vi "Handle Camera Configuration.vi"(9 "CameraNameRef":refnum<vi>, 10 "Camera File Name":string="Camera", 11 "ClusterRef":refnum<vi>) -> ()   [LabVIEW 2016]
uses:
  <vilib>/Utility/config.llb/NI_LVConfig.lvlib
  <vilib>/Rock Robotics/Network Tables/Make Table Operation.ctl
  <vilib>/Utility/config.llb/Read Key (I32).vi
  <vilib>/Utility/config.llb/Read Key (String).vi
  <vilib>/Utility/config.llb/Write Key (I32).vi
  <vilib>/Utility/config.llb/Write Key (String).vi
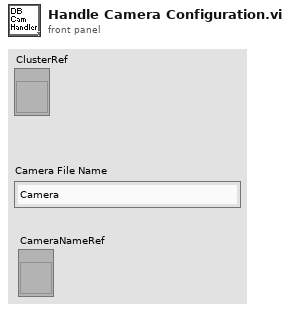
[diagram p1: front panel]
types:
  T1 = typedef "WPI_CameraDevRef.ctl" = cluster{"Camera Address":string, "CameraStatus":errorcluster}
  T2 = typedef "NI_LVConfig.lvlib/Config Data RefNum.ctl" = refnum<k1>
  T3 = cluster{"value":i32, "value":i32, "index":i32, bool}
  T4 = typedef "Make Table Operation.ctl" = enum16{"Get or Add Field", "Get Field or Add Temp", "Replace Temp ID", "Get Field ID - No Add", "Get Table Field IDs", "Get Field ID Info", "Move Field to Temp", "Validate", "Remove Field", "Remove All"}
  T5 = cluster{"Frame Rate":i32, "Compression":i32, "Size":u16, "DB Camera Config":bool}
  T6 = typedef "Field ID.ctl" = i32
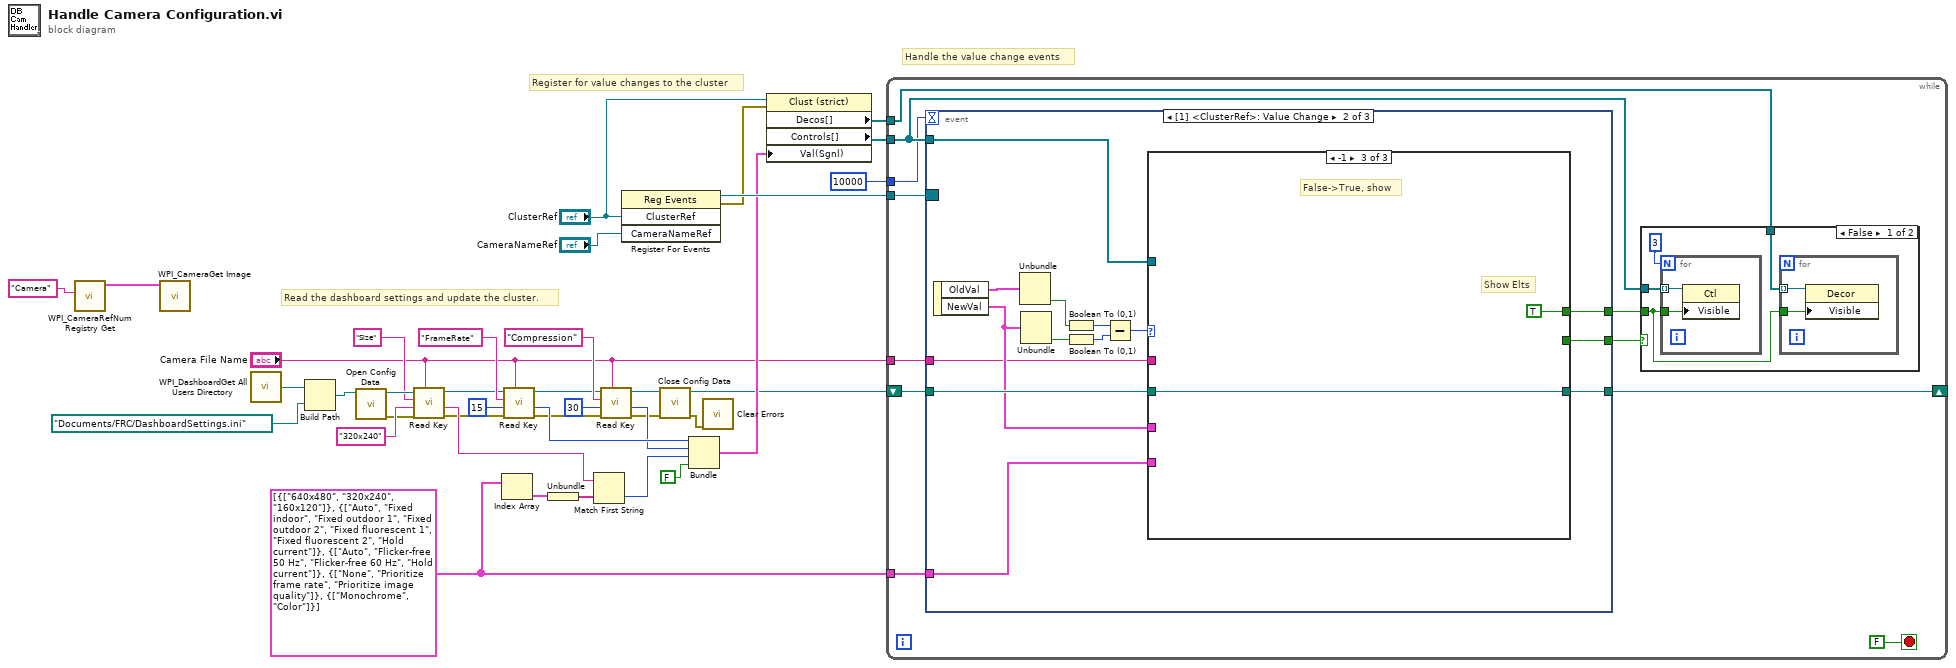
[diagram p0: block diagram]
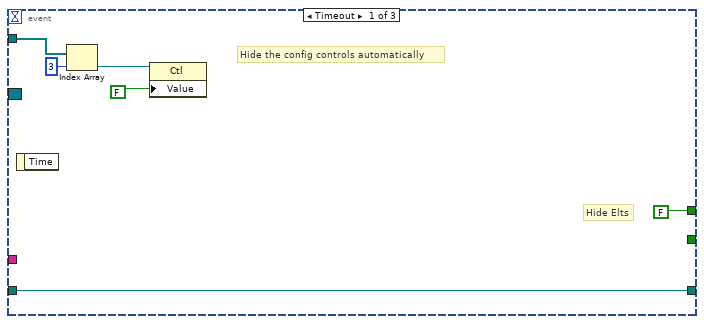
[diagram p3: hidden frame]
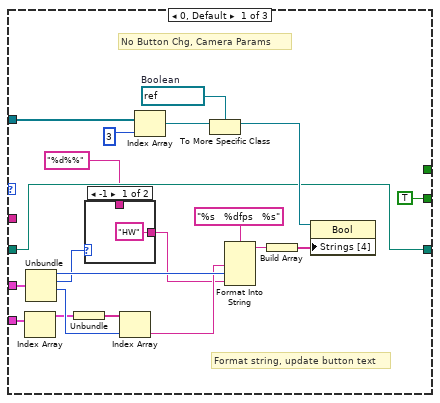
[diagram p4: hidden frame]
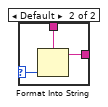
[diagram p5: hidden frame]
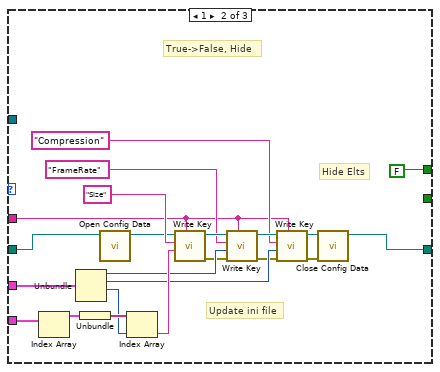
[diagram p6: hidden frame]
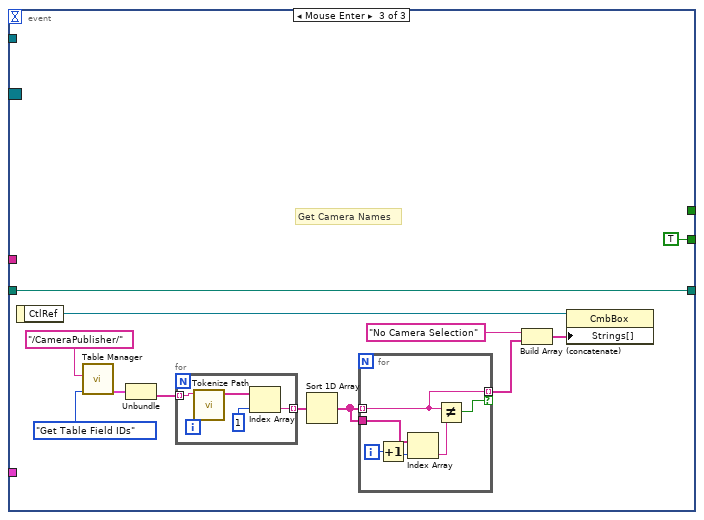
[diagram p7: hidden frame]
diagram:
  w17 = cluster{string[]}[] [{["640x480", "320x240", "160x120"]}, {["Auto", "Fixed indoor", "Fixed outdoor 1", "Fixed outdoor 2", "Fixed fluorescent 1", "Fixed fluorescent 2", "Hold current"]}, {["Auto", "Flicker-free 50 Hz", "Flicker-free 60 Hz", "Hold current"]}, {["None", "Prioritize frame rate", "Prioritize image quality"]}, {["Monochrome", "Color"]}]
  # "Handle the value change events"
  # "Register for value changes to the cluster"
  # "Read the dashboard settings and update the cluster."
  n1 = call <vilib>:"WPI_CameraRefNum Registry Get.vi"("refnum name"="Camera") -> ("CameraDevRef"=w1:T1)  [unwired: 9 in, 1 out]
  n2 = call <vilib>:"WPI_CameraGet Image.vi"("CameraDevRef"=w1) -> ()  [unwired: 8 in, 3 out]
  n3 = call <vilib>:"WPI_DashboardGet All Users Directory.vi"() -> ("All User Path"=w35:path)
  n4 = Build Path(base path=w35, name or relative path=path "Documents/FRC/DashboardSettings.ini") -> (appended path=w34:path)
  n5 = call <vilib>:"Open Config Data.vi"("configuration file path"=w34) -> ("error out"=w10:errorcluster, "refnum"=w33:T2)  [unwired: 8 in, 1 out]
  n6 = call-poly <vilib>:"Read Key.vi"("section"="Camera File Name", "error in (no error)"=w10, "default value"="320x240", "key"="Size", "refnum"=w33) -> ("error out"=w9:errorcluster, "value"=w21:string, "refnum out"=w25:T2)  [unwired: 1 in, 3 out]
  n7 = Index Array(array=w17) -> (element=w23:cluster{string[]})  [unwired: 1 in]
  n8 = call-poly <vilib>:"Read Key.vi"("section"="Camera File Name", "error in (no error)"=w9, "default value"=15, "key"="FrameRate", "refnum"=w25) -> ("error out"=w8:errorcluster, "value"=w19:i32, "refnum out"=w24:T2)  [unwired: 4 out]
  n9 = Unbundle(w23) -> (w22:string[])
  n10 = Match First String(2:w22, 3:w21) -> (0:w20:i32)  [unwired: 1 out]
  n11 = call-poly <vilib>:"Read Key.vi"("section"="Camera File Name", "error in (no error)"=w8, "default value"=30, "key"="Compression", "refnum"=w24) -> ("error out"=w5:errorcluster, "value"=w18:i32, "refnum out"=w7:T2)  [unwired: 4 out]
  n12 = register-events("ClusterRef", "CameraNameRef") -> (reference out=w38:refnum<event-registration>, error out=w15:errorcluster)  [unwired: 2 in]
  n13 = call <vilib>:"Close Config Data.vi"("error in (no error)"=w5, "refnum"=w7) -> ("error out"=w4:errorcluster, "file path"=w6:path)  [unwired: 1 in, 7 out]
  n14 = Bundle("value"=w19, "value"=w18, "index"=w20, FALSE) -> (w14:T3)  [unwired: 1 out]
  n15 = call <vilib>:"Clear Errors.vi"("error in (no error)"=w4) -> ()  [unwired: 5 in, 2 out]
  n16 = property class="Clust (strict)"(reference="ClusterRef", error in=w15, "Val(Sgnl)"=w14) -> ("Decos[]"=w12:refnum<vi>[], "Controls[]"=w36:refnum<vi>[])  [unwired: 2 out]
  n17 = while {
    tunnel: w38 -> [w49]
    tunnel: w36 -> [w41]
    shift-right: [w47] -> _
    shift-left: w6 -> [w48]
    tunnel: w17 -> [w46]
    tunnel: "Camera File Name" -> [w44]
    tunnel: w12 -> [w40]
    tunnel: 10000 -> [w39]
    stop <- FALSE stop-if-true
    n18 = event shown="[1] <ClusterRef>: Value Change" {
      selector: w49 -> [_ _ _]
      dyn-events: _ -> [_ _ _]
      timeout: w39 -> [_ _ _]
      tunnel: w48 -> [w62 w71 w135]
      tunnel: [w62 w67 w135] -> w47
      tunnel: w46 -> [_ w69 _]
      tunnel: w41 -> [w61 w68 _]
      tunnel: w44 -> [_ w66 _]
      tunnel: [FALSE w65 _] -> w42
      tunnel: [_ w64 TRUE] -> w43
      event Timeout {
        # "Hide Elts"
        # "Hide the config controls automatically"
        n19 = event-data() -> ()  [unwired: 1 in, 1 out]
        n20 = Index Array(array=w61, index=3) -> (element=w59:refnum<vi>)
        n21 = property class="Ctl"(reference=w59, "Value"=FALSE) -> ()  [unwired: 1 in, 2 out]
      }
      event Value Change {
        n22 = event-data() -> ("OldVal"=w73:T5, "NewVal"=w70:T5)  [unwired: 1 in]
        n23 = Unbundle(w73) -> ("DB Camera Config"=w77:bool)  [unwired: 3 out]
        n24 = Unbundle(w70) -> ("DB Camera Config"=w76:bool)  [unwired: 3 out]
        n25 = Boolean To (0,1)(Boolean=w77) -> (0, 1=w74:i16)
        n26 = Boolean To (0,1)(Boolean=w76) -> (0, 1=w75:i16)
        n27 = Subtract(x=w74, y=w75) -> (x-y=w72:i16)
        n28 = case shown="-1" w72 {
          tunnel: [_ FALSE TRUE] -> w65
          tunnel: [TRUE _ _] -> w64
          tunnel: w71 -> [w81 w104 w124]
          tunnel: w70 -> [w89 w113 _]
          tunnel: w69 -> [w88 w109 _]
          tunnel: w68 -> [w87 _ _]
          tunnel: [w81 w102 w124] -> w67
          tunnel: w66 -> [_ w108 _]
          frame 0, Default {
            w84 = refnum<vi> refnum  # Boolean
            # "Format string, update button text"
            # "No Button Chg, Camera Params"
            n29 = Index Array(array=w88) -> (element=w92:cluster{string[]})  [unwired: 1 in]
            n30 = Unbundle(w89) -> ("Frame Rate"=w96:i32, "Compression"=w78:i32, "Size"=w94:u16)  [unwired: 1 out]
            n31 = Unbundle(w92) -> (w93:string[])
            n32 = case shown="-1" w78 {
              selector: w78 -> [_ w99]
              tunnel: "%d%%" ("format string") -> [_ w101]
              tunnel: ["HW" ("format string") w100] -> w79
              frame -1 {
              }
              frame Default {
                n33 = Format Into String(format string=w101, w99) -> (resulting string=w100:string)  [unwired: 2 in, 1 out]
              }
            }
            n34 = Index Array(array=w93, index=w94) -> (element=w95:string)
            n35 = Index Array(array=w87, index=3) -> (element=w85:refnum<vi>)
            n36 = To More Specific Class(target class=w84, reference=w85) -> (specific class reference=w83:refnum<vi>)  [unwired: 1 in, 1 out]
            n37 = Format Into String(format string="%s   %dfps   %s", w95, w96, w79) -> (resulting string=w91:string)  [unwired: 2 in, 1 out]
            n38 = Build Array(w91) -> (w82:string[])
            n39 = property class="Bool"(reference=w83, "Strings [4]"=w82) -> ()  [unwired: 1 in, 2 out]
          }
          frame 1 {
            # "Update ini file"
            # "Hide Elts"
            # "True->False, Hide"
            n40 = Index Array(array=w109) -> (element=w117:cluster{string[]})  [unwired: 1 in]
            n41 = Unbundle(w113) -> ("Frame Rate"=w112:i32, "Compression"=w111:i32, "Size"=w110:u16)  [unwired: 1 out]
            n42 = Unbundle(w117) -> (w116:string[])
            n43 = call <vilib>:"Open Config Data.vi"("configuration file path"=w104) -> ("refnum"=w103:T2)  [unwired: 8 in, 2 out]
            n44 = Index Array(array=w116, index=w110) -> (element=w115:string)
            n45 = call-poly <vilib>:"Write Key.vi"("section"=w108, "value"=w115, "key"="Size", "refnum"=w103) -> ("error out"=w107:errorcluster, "refnum out"=w122:T2)  [unwired: 2 in, 4 out]
            n46 = call-poly <vilib>:"Write Key.vi"("section"=w108, "error in (no error)"=w107, "value"=w112, "key"="FrameRate", "refnum"=w122) -> ("error out"=w106:errorcluster, "refnum out"=w121:T2)  [unwired: 5 out]
            n47 = call-poly <vilib>:"Write Key.vi"("section"=w108, "error in (no error)"=w106, "value"=w111, "key"="Compression", "refnum"=w121) -> ("error out"=w105:errorcluster, "refnum out"=w114:T2)  [unwired: 5 out]
            n48 = call <vilib>:"Close Config Data.vi"("error in (no error)"=w105, "refnum"=w114) -> ("file path"=w102:path)  [unwired: 1 in, 8 out]
          }
          frame -1 {
            # "Show Elts"
            # "False->True, show"
          }
        }
      }
      event Mouse Enter {
        # "Get Camera Names"
        n49 = event-data() -> ("CtlRef"=w137:refnum<vi>)  [unwired: 1 in]
        n50 = call <vilib>:"Table Manager.vi"("Operation"=Make_Table_Operation."Get Table Field IDs", "Entry Name"="/CameraPublisher/") -> ("Entries"=w132:cluster{"Entry IDs":T6[], "Names":string[]})  [unwired: 6 in, 3 out]
        n51 = Unbundle(w132) -> ("Names"=w129:string[])  [unwired: 1 out]
        n52 = for {
          tunnel: w129 -> [w147] mode=indexing
          tunnel: [w144] -> w128 mode=indexing
          n53 = call <vilib>:"Tokenize Path.vi"("Name"=w147) -> ("Array"=w146:string[])  [unwired: 10 in]
          n54 = Index Array(array=w146, index=1) -> (element=w144:string)
        }
        n55 = Sort 1D Array(array=w128) -> (sorted array=w127:string[])
        n56 = for {
          tunnel: w127 -> [w139] mode=indexing
          tunnel: w127 -> [w141]
          tunnel: [w139] -> w126 mode=indexing if=w138
          i -> [w143]
          n57 = Increment(x=w143) -> (x+1=w142:i32)
          n58 = Index Array(array=w141, index=w142) -> (element=w140:string)
          n59 = Not Equal?(x=w139, y=w140) -> (x != y?=w138:bool)
        }
        n60 = Build Array (concatenate)("No Camera Selection", w126) -> (w130:string[])
        n61 = property class="CmbBox"(reference=w137, "Strings[]"=w130) -> ()  [unwired: 1 in, 2 out]
      }
    }
    n62 = case shown="False" w43 {
      tunnel: w41 -> [w53 _]
      tunnel: w42 -> [w50 _]
      tunnel: w40 -> [w51 _]
      frame False {
        n63 = for {
          N: 3 -> [_]
          tunnel: w53 -> [w57] mode=indexing
          tunnel: w50 -> [w56]
          n64 = property class="Ctl"(reference=w57, "Visible"=w56) -> ()  [unwired: 1 in, 2 out]
        }
        n65 = for {
          tunnel: w51 -> [w55] mode=indexing
          tunnel: w50 -> [w54]
          n66 = property class="Decor"(reference=w55, "Visible"=w54) -> ()  [unwired: 1 in, 2 out]
        }
      }
      frame True {
      }
    }
  }
